vi "temp_test.vi"() -> ()   [LabVIEW 2021]
uses:
  <vilib>/myRIO/Common/Instrument Driver Framework/Utilities/vis/Validate Channels.vi
  <vilib>/myRIO/Common/Instrument Driver Framework/myRIO v1.0/I2C/vis/myRIO v1.0 Reserve I2C.vi
  <vilib>/myRIO/Common/Instrument Driver Framework/myRIO v1.0/I2C/vis/myRIO v1.0 Build MUX Configuration I2C.vi
  <vilib>/myRIO/Common/Instrument Driver Framework/myRIO v1.0/Resource Manager/vis/myRIO v1.0 Reserve Channel List.vi
  <vilib>/myRIO/Common/Instrument Driver Framework/myRIO v1.0/Resource Manager/vis/myRIO v1.0 Create Configuration List.vi
  <vilib>/myRIO/Common/Instrument Driver Framework/myRIO v1.0/Resource Manager/vis/myRIO v1.0 Reserve Channel.vi
  <vilib>/myRIO/Common/Instrument Driver Framework/myRIO v1.0/Resource Manager/vis/myRIO v1.0 Unreserve Channel.vi
  <vilib>/myRIO/Common/Instrument Driver Framework/myRIO v1.0/Resource Manager/vis/myRIO v1.0 Build Mutex Name.vi
  <vilib>/Utility/error.llb/Error Cluster From Error Code.vi
  <vilib>/myRIO/Common/Instrument Driver Framework/myRIO v1.0/I2C/vis/myRIO v1.0 Configure I2C.vi
  <vilib>/Utility/VariantDataType/GetNumericInfo.vi
  <vilib>/myRIO/Common/Instrument Driver Framework/myRIO v1.0/myRIO v1.1 Open.vi
  <vilib>/myRIO/Common/Instrument Driver Framework/Utilities/vis/IO Manager.vi
  <vilib>/myRIO/Common/Instrument Driver Framework/Utilities/vis/Configuration Manager.vi
  <vilib>/myRIO/Common/Instrument Driver Framework/myRIO v1.0/Resource Manager/vis/myRIO v1.0 Configure IO.vi
  <vilib>/myRIO/Common/Instrument Driver Framework/myRIO v1.0/myRIO v1.0 Close.vi
  <vilib>/myRIO/Common/Instrument Driver Framework/myRIO v1.0/I2C/vis/myRIO v1.0 Write I2C.vi
  <vilib>/myRIO/Common/Instrument Driver Framework/myRIO v1.0/I2C/vis/myRIO v1.0 Read I2C.vi
  <vilib>/myRIO/Common/Instrument Driver Framework/myRIO v1.0/DIO/vis/myRIO v1.0 Read DIO.vi
  <vilib>/myRIO/Instrument Drivers/Onboard IO/I2C/typedefs/I2C Reference.ctl
  <vilib>/myRIO/Instrument Drivers/Onboard IO/I2C/typedefs/I2C Configuration.ctl
  <vilib>/myRIO/Instrument Drivers/Onboard IO/I2C/typedefs/I2C Transfer Rate.ctl
  <vilib>/myRIO/Common/Instrument Driver Framework/myRIO v1.0/I2C/typedefs/I2C Channels Enum.ctl
  <vilib>/myRIO/Common/Instrument Driver Framework/Utilities/typedefs/myRIO Generic Hardware Reference.ctl
  <vilib>/myRIO/Common/Instrument Driver Framework/Utilities/typedefs/myRIO v1.0 Reference.ctl
  <vilib>/myRIO/Common/Instrument Driver Framework/Utilities/typedefs/Generic FPGA Reference.ctl
  <vilib>/myRIO/Common/Instrument Driver Framework/Utilities/typedefs/Hardware Version Enum.ctl
  <vilib>/myRIO/Instrument Drivers/Onboard IO/I2C/typedefs/I2C User Configuration.ctl
  <vilib>/myRIO/Instrument Drivers/Onboard IO/I2C/vis/Write Read.vi
  <vilib>/userDefined/High Color/nirio_resource_hc.ctl
  <vilib>/myRIO/Common/Instrument Driver Framework/myRIO v1.0/I2C/vis/myRIO v1.1 Open I2C.vi
  <vilib>/myRIO/Common/Instrument Driver Framework/Utilities/vis/Is FPGA Ref Available.vi
  <vilib>/myRIO/Instrument Drivers/Onboard IO/I2C/vis/Write.vi
  <vilib>/myRIO/Instrument Drivers/Onboard IO/I2C/I2C.lvlib
  <vilib>/myRIO/Instrument Drivers/Onboard IO/DIO/DIO.lvlib
  <vilib>/myRIO/Express VI/Onboard IO/I2C/I2C Express VI.xnode
  <vilib>/myRIO/Instrument Drivers/Onboard IO/I2C/vis/myRIO I2C Open.xnode
panel:
  in  "stop":bool
  out "Temperature ?":dbl(slide) scale=0.0..100.0
  out "Ta":u8[](array[numeric])
  out "Alert":bool
  out "Thyst (hysteresis)":u8[](array[numeric]) format="%x"
  out "TSet":u8[](array[numeric]) format="%x"
  out "Config":u8[](array[numeric])
  # "https://www.youtube.com/watch?v=1Oib10sojds"
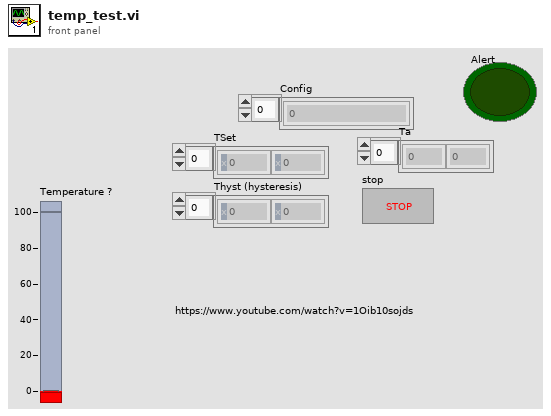
[diagram p1: front panel]
types:
  T1 = typedef "I2C.lvlib/I2C User Configuration.ctl" = cluster{"I2C Transfer Rate":T2}
  T2 = typedef "I2C.lvlib/I2C Transfer Rate.ctl" = enum16{"Standard mode (100 kbps)", "Fast mode (400 kbps)"}
  T3 = typedef "I2C.lvlib/I2C Reference.ctl" = cluster{"myRIO Reference":T4, "I2C Channels Enum":T8, "I2C Configuration":T9}
  T4 = typedef "myRIO Generic Hardware Reference.ctl" = cluster{"myRIO Model":T5, "myRIO Hardware Reference":T6}
  T5 = typedef "Hardware Version Enum.ctl" = enum16{"Unknown", "myRIO-1900", "myRIO-1950", "roboRIO", "NI ELVIS RIO CM", "ELVIS III"}
  T6 = typedef "myRIO v1.0 Reference.ctl" = cluster{"Generic FPGA Reference":T7, "Allow multiple opens":bool}
  T7 = typedef "Generic FPGA Reference.ctl" = refnum<k20>
  T8 = typedef "I2C Channels Enum.ctl" = enum16{"Not Connected", "A/I2C", "B/I2C", "I2C/I2C"}
  T9 = typedef "I2C.lvlib/I2C Configuration.ctl" = cluster{"I2C Transfer Rate":T2}
  T10 = typedef "DIO.lvlib/DIO Reference.ctl" = cluster{"myRIO Reference":T4, "DIO Channels List":T11}
  T11 = typedef "DIO Channels List.ctl" = T12[]
  T12 = typedef "DIO Channels Enum.ctl" = enum16{"Not Connected", "C/DIO0", "C/DIO1", "C/DIO2", "C/DIO3", "C/DIO4", "C/DIO5", "C/DIO6", "C/DIO7", "A/DIO0", "A/DIO1", "A/DIO2", "A/DIO3", "A/DIO4", "A/DIO5", "A/DIO6", "A/DIO7", "A/DIO8", "A/DIO9", "A/DIO10", "A/DIO11", "A/DIO12", "A/DIO13", "A/DIO14", "A/DIO15", "A/DIO16", "A/DIO17", "A/DIO18", "A/DIO19", "B/DIO0", "B/DIO1", "B/DIO2", "B/DIO3", "B/DIO4", "B/DIO5", "B/DIO6", "B/DIO7", "B/DIO8", "B/DIO9", "B/DIO10", "B/DIO11", "B/DIO12", "B/DIO13", "B/DIO14", "B/DIO15", "B/DIO16", "B/DIO17", "B/DIO18", "B/DIO19", "LED0", "LED1", "LED2", "LED3", "Button0", "DIO/DIO0", "DIO/DIO1", "DIO/DIO2", "DIO/DIO3", "DIO/DIO4", "DIO/DIO5", "DIO/DIO6", "DIO/DIO7", "DIO/DIO8", "DIO/DIO9", "SPI/CS0", "SPI/CS1", "SPI/CS2", "SPI/CS3", "LED RADIO (Green)", "LED RADIO (Red)", "LED COMM (Green)", "LED COMM (Red)", "LED MODE (Green)", "LED MODE (Red)"}
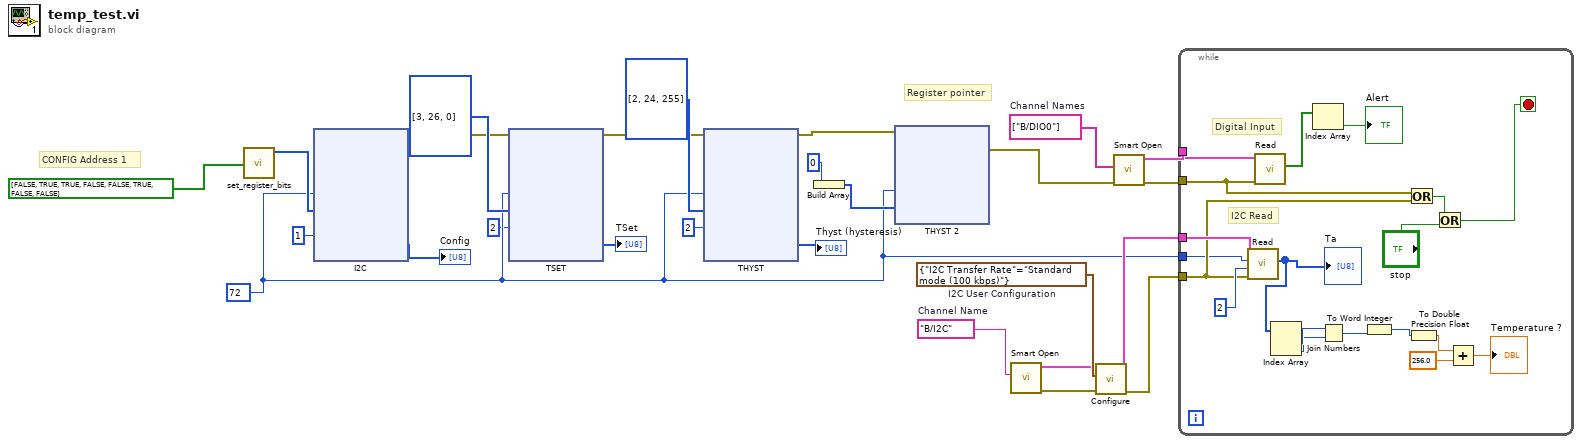
[diagram p0: block diagram]
diagram:
  w9 = tag[] ["B/DIO0"]  # Channel Names
  w12 = T1 {"I2C Transfer Rate"=enum."Standard mode (100 kbps)"}  # I2C User Configuration
  w13 = tag "B/I2C"  # Channel Name
  w3 = u8 72 ("Slave Address (7-bit)")
  # "Register pointer"
  # "CONFIG Address 1"
  n1 = call "set_register_bits.vi"("Array in"=bool[] [FALSE, TRUE, TRUE, FALSE, FALSE, TRUE, FALSE, FALSE]) -> ("Array out"=w25:u8[])  [unwired: 10 in]
  n2 = xnode "I2C"("Slave Address (7-bit)"=w3, "Bytes to Write"=w25, "Byte Count"=u32 1) -> ("Bytes Read"=→"Config":u8[], "error out"=w19:errorcluster)  [unwired: 1 in]
  n3 = xnode "TSET"("Slave Address (7-bit)"=w3, "Bytes to Write"=u8[] [3, 26, 0], "Byte Count"=u32 2, "error in (no error)"=w19) -> ("Bytes Read"=→"TSet":u8[], "error out"=w18:errorcluster)
  n4 = xnode "THYST"("Slave Address (7-bit)"=w3, "Bytes to Write"=u8[] [2, 24, 255], "Byte Count"=u32 2, "error in (no error)"=w18) -> ("Bytes Read"=→"Thyst (hysteresis)":u8[], "error out"=w17:errorcluster)
  n5 = Build Array(0) -> (w15:i32[])
  n6 = xnode "THYST 2"("Slave Address (7-bit)"=w3, "Bytes to Write"=w15, "error in (no error)"=w17) -> ("error out"=w6:errorcluster)
  n7 = call <vilib>:"Smart Open.vi"("Channel Name"=w13) -> ("error out"=w10:errorcluster, "I2C Ref Out"=w11:T3)  [unwired: 9 in]
  n8 = call <vilib>:"Configure.vi"("error in (no error)"=w10, "I2C User Configuration"=w12, "I2C Ref In"=w11) -> ("error out"=w5:errorcluster, "I2C Ref Out"=w4:T3)  [unwired: 7 in]
  n9 = call <vilib>:"Smart Open.vi"("error in (no error)"=w6, "Channel Names"=w9) -> ("error out"=w8:errorcluster, "DIO Ref Out"=w7:T10)  [unwired: 8 in]
  n10 = while {
    tunnel: w8 -> [w32]
    tunnel: w7 -> [w43]
    tunnel: w5 -> [w31]
    tunnel: w4 -> [w41]
    tunnel: w3 -> [w27]
    stop <- w28 stop-if-true
    # "I2C Read"
    # "Digital Input"
    n11 = call <vilib>:"Read.vi"("error in (no error)"=w31, "Byte Count"=u32 2, "Slave Address (7-bit)"=w27, "I2C Ref In"=w41) -> ("Bytes Read"=w40:u8[])  [unwired: 4 in, 2 out]
    "Ta" <- w40
    n12 = call <vilib>:"Read.vi"("error in (no error)"=w32, "DIO Ref In"=w43) -> ("Values"=w44:bool[])  [unwired: 7 in, 2 out]
    n13 = Index Array(array=w40) -> (element #1=w39:u8, element #2=w38:u8)  [unwired: 2 in]
    n14 = Index Array(array=w44) -> (element=→"Alert":bool)  [unwired: 1 in]
    n15 = Join Numbers(hi=w39, lo=w38) -> ((hi.lo)=w37:u16)
    n16 = To Word Integer(number=w37) -> (16bit integer=w36:i16)
    n17 = Or(x=w32, y=w31) -> (x .or. y?=w30:bool)
    n18 = To Double Precision Float(number=w36) -> (double precision float=w35:dbl)
    n19 = Or(x=w30, y="stop") -> (x .or. y?=w28:bool)
    n20 = Add(x=w35, y=256.0) -> (x+y=→"Temperature ?":dbl)
  }
